vi "MUX_example.vi"() -> ()   [LabVIEW 2013]
doc: "Equipment required: a multiplexer card ( 34921 - 34925 ) in slot 2, and internal DMM present and enabled in the 34980.\n\nThe example shows how to configure multiple channels for different functions and different measurement ranges on those functions (besides auto-range). You need to use Configure + Init + Fetch as shown here when you wish to:\n -- measure different functions in a single scan\n -- specify triggering other than the default ( immediate)\n -- want to change the NPLC or Aperture time for faster reading rates.\n\n In contrast, the 'Measure' VIs found in the Data section force a trigger source of immediate and the same function measurement on the scanned channels."
panel:
  in  "Show Units in Data":bool
  in  "Show Channel In Data":bool
  in  "VISA resource name":refnum<visa-resource-name>
  out "Output Results":string[](array[string])
  out "Scan Size":dbl
  out "VISA/Instrument Errors":errorcluster
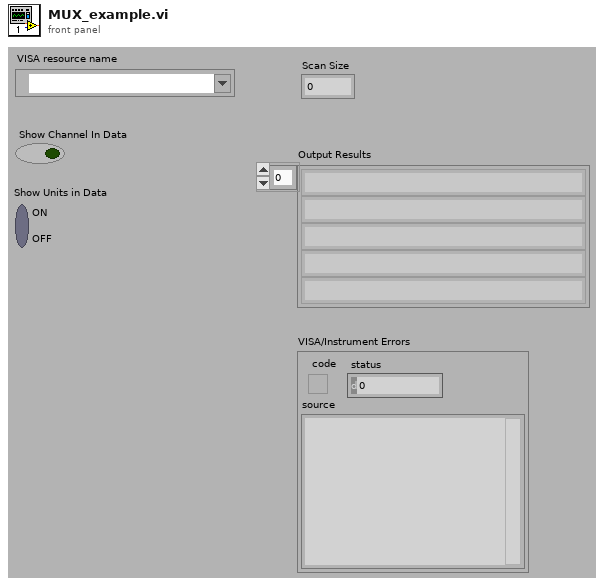
[diagram p1: front panel]
types:
  T1 = enum16{"Bus", "Immediate", "External", "Alarm 1", "Alarm 2", "Alarm 3", "Alarm 4", "Timer"}
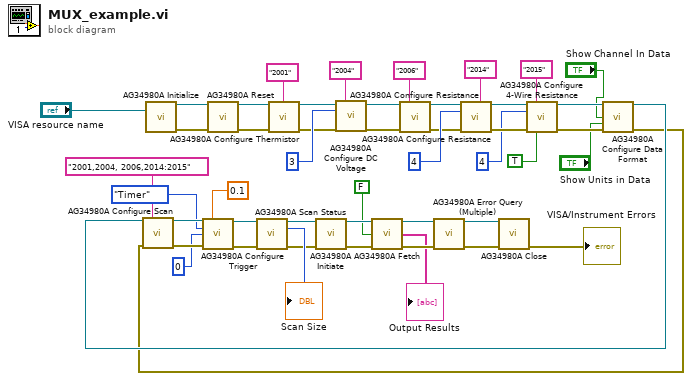
[diagram p0: block diagram]
diagram:
  n1 = call "AG34980A Initialize.vi"("VISA resource name"="VISA resource name") -> ("VISA session"=w48:refnum<visa-resource-name>, "error out"=w47:errorcluster)  [unwired: 13 in]
  n2 = call "AG34980A Reset.vi"("VISA resource name"=w48, "error in (no error)"=w47) -> ("VISA resource name out"=w34:refnum<visa-resource-name>, "error out"=w33:errorcluster)  [unwired: 12 in]
  n3 = call "AG34980A Configure Thermistor.vi"("VISA resource name"=w34, "Channel List(empty)"="2001", "error in (no error)"=w33) -> ("VISA resource name out"=w32:refnum<visa-resource-name>, "error out"=w31:errorcluster)  [unwired: 11 in]
  n4 = call "AG34980A Configure DC Voltage.vi"("VISA resource name"=w32, "Channel List(empty)"="2004", "Range (5:Auto)"=3, "error in (no error)"=w31) -> ("VISA resource name out"=w45:refnum<visa-resource-name>, "error out"=w44:errorcluster)  [unwired: 10 in]
  n5 = call "AG34980A Configure Resistance.vi"("VISA resource name"=w45, "Channel List(empty)"="2006", "error in (no error)"=w44) -> ("VISA resource name out"=w22:refnum<visa-resource-name>, "error out"=w21:errorcluster)  [unwired: 11 in]
  n6 = call "AG34980A Configure Resistance.vi"("VISA resource name"=w22, "Channel List(empty)"="2014", "Range (7:Auto)"=4, "error in (no error)"=w21) -> ("VISA resource name out"=w42:refnum<visa-resource-name>, "error out"=w41:errorcluster)  [unwired: 10 in]
  n7 = call "AG34980A Configure 4-Wire Resistance.vi"("VISA resource name"=w42, "Channel List(empty)"="2015", "Range (7:Auto)"=4, "error in (no error)"=w41, "Offset Compensation (F:Off)"=TRUE) -> ("VISA resource name out"=w6:refnum<visa-resource-name>, "error out"=w4:errorcluster)  [unwired: 9 in]
  n8 = call "AG34980A Configure Data Format.vi"("VISA resource name"=w6, "Channel Enable (F:Off)"="Show Channel In Data", "Unit Enable (F:Off)"="Show Units in Data", "error in (no error)"=w4) -> ("VISA resource name out"=w5:refnum<visa-resource-name>, "error out"=w3:errorcluster)  [unwired: 10 in]
  n9 = call "AG34980A Configure Scan.vi"("VISA resource name"=w5, "Scan List(empty)"="2001,2004, 2006,2014:2015", "error in (no error)"=w3) -> ("VISA resource name out"=w20:refnum<visa-resource-name>, "error out"=w19:errorcluster)  [unwired: 11 in]
  n10 = call "AG34980A Configure Trigger.vi"("VISA resource name"=w20, "Trigger Timer Value (0 sec)"=0.1, "Trigger Source (1:Immediate)"=T1."Timer", "Max Trigger Count (0:Specify Count)"=0, "error in (no error)"=w19) -> ("VISA resource name out"=w29:refnum<visa-resource-name>, "error out"=w28:errorcluster)  [unwired: 9 in]
  n11 = call "AG34980A Scan Status.vi"("VISA resource name"=w29, "error in (no error)"=w28) -> ("VISA resource name out"=w26:refnum<visa-resource-name>, "Scan Size"=→"Scan Size":u32, "error out"=w25:errorcluster)  [unwired: 10 in, 1 out]
  n12 = call "AG34980A Initiate.vi"("VISA resource name"=w26, "error in (no error)"=w25) -> ("VISA resource name out"=w24:refnum<visa-resource-name>, "error out"=w17:errorcluster)  [unwired: 12 in]
  n13 = call "AG34980A Fetch.vi"("VISA resource name"=w24, "Numbers Only (T:On)"=FALSE, "error in (no error)"=w17) -> ("VISA resource name out"=w15:refnum<visa-resource-name>, "Output Data"=→"Output Results":string[], "error out"=w16:errorcluster)  [unwired: 9 in, 1 out]
  n14 = call "AG34980A Error Query (Multiple).vi"("VISA resource name"=w15, "error in (no error)"=w16) -> ("VISA resource name out"=w13:refnum<visa-resource-name>, "error out"=w14:errorcluster)  [unwired: 10 in, 2 out]
  n15 = call "AG34980A Close.vi"("VISA resource name"=w13, "error in (no error)"=w14) -> ("error out"=→"VISA/Instrument Errors":errorcluster)  [unwired: 13 in]
